vi "loop2.vi"() -> ()   [LabVIEW 2010]
uses:
  <vilib>/Utility/file.llb/Write To Spreadsheet File (DBL).vi
panel:
  out "Array":dbl[](array[numeric])
  in  "Path":path
  out "XY Graph 2":cluster{dbl[], dbl[]}(graph)
  out "XY Graph":cluster{dbl[], dbl[]}(graph)
  out "error out":errorcluster
  in  "error in (no error)":errorcluster
  out "Numeric":dbl format="%.2f"
  in  "Start":dbl format="%.2f"
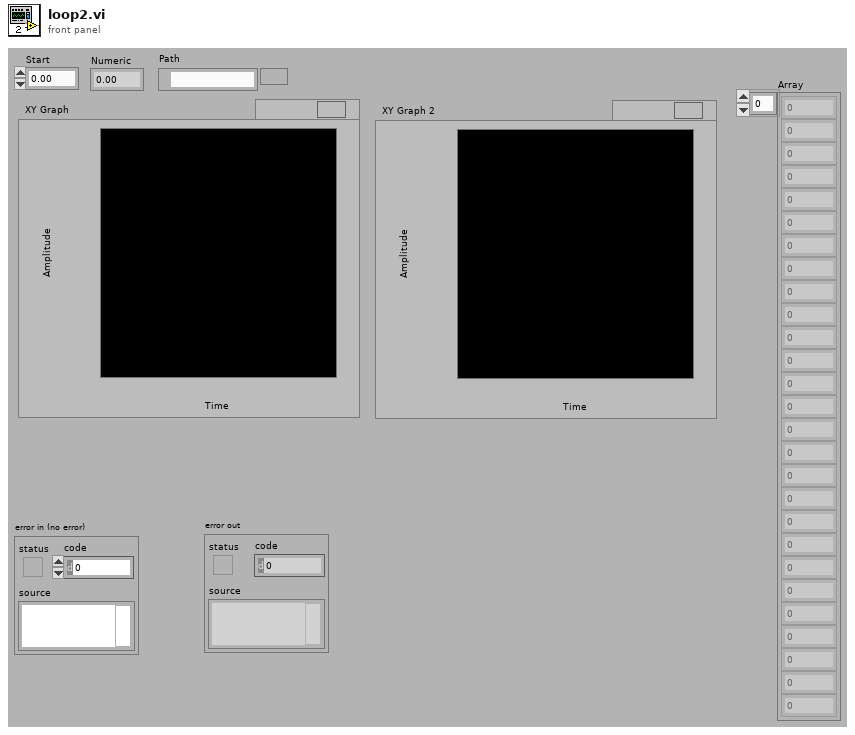
[diagram p1: front panel]
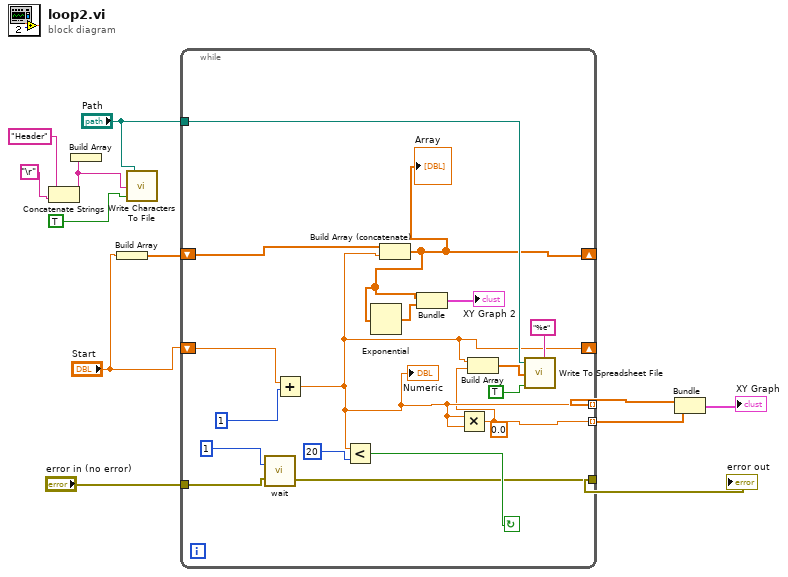
[diagram p0: block diagram]
diagram:
  n1 = Concatenate Strings("Header", "\r") -> (w2:string)
  n2 = Build Array(w2) -> ()  [unwired: 1 out]
  n3 = Build Array("Start") -> (w6:dbl[])
  n4 = call <vilib>:"Write Characters To File.vi"("append to file? (new file:F)"=TRUE, "character string"=w2, "file path (dialog if empty)"="Path") -> ()  [unwired: 2 in, 1 out]
  n5 = while {
    tunnel: "error in (no error)" -> [w27]
    tunnel: [w26] -> w11
    shift-right: [w16] -> _
    shift-left: "Start" -> [w23]
    tunnel: [w16] -> w10 mode=indexing
    tunnel: [w15] -> w9 mode=indexing
    shift-right: [w13] -> _
    shift-left: w6 -> [w22]
    tunnel: "Path" -> [w19]
    stop <- w28 continue-if-true
    (unwired) 0.0
    n6 = call "wait.vi"("error in"=w27, "Wartezeit in Sek"=1) -> ("error out"=w26:errorcluster)  [unwired: 1 in]
    n7 = Add(x=w23, y=1) -> (x+y=w16:dbl)
    "Numeric" <- w16
    n8 = Less?(x=w16, y=20) -> (x < y?=w28:bool)
    n9 = Build Array (concatenate)(w22, w16) -> (w13:dbl[])
    "Array" <- w13
    n10 = Exponential(1:w13) -> (0:w20:dbl[])
    n11 = Bundle(w13, w20) -> (→"XY Graph 2":cluster{dbl[], dbl[]})  [unwired: 1 in]
    n12 = Multiply(x=w16, y=w16) -> (x*y=w15:dbl)
    n13 = Build Array(w16, w15) -> (w14:dbl[])
    n14 = call-poly <vilib>:"Write To Spreadsheet File.vi"("format (%.3f)"="%e", "append to file? (new file:F)"=TRUE, "1D data"=w14, "file path (dialog if empty)"=w19) -> ()  [unwired: 4 in, 1 out]
  }
  "error out" <- w11
  n15 = Bundle(w10, w9) -> (→"XY Graph":cluster{dbl[], dbl[]})  [unwired: 1 in]
